vi "SendHRS.vi"(8 "error in (no error)":errorcluster, 10 "HRS data":u32[](array[numeric]), 11 "Database ref":refnum<k24>) -> (0 "error out":errorcluster)   [LabVIEW 2015]
uses:
  C:/Users/Bartek/Desktop/NORDIC Labview GUI/DLLs/NordicDatabaseDLL.dll
  DLLs/NordicDatabaseDLL.dll
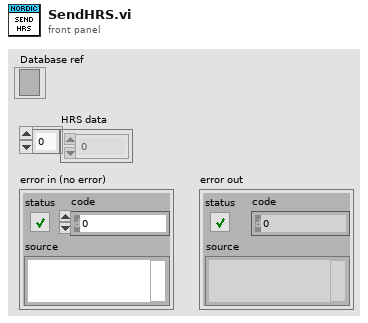
[diagram p1: front panel]
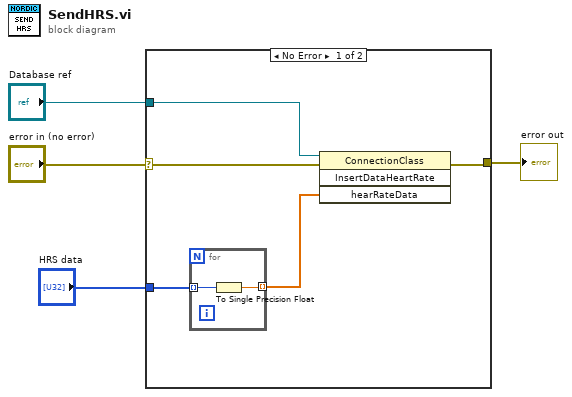
[diagram p0: block diagram]
diagram:
  n1 = case shown="No Error" "error in (no error)" {
    selector: "error in (no error)" -> [w8 w12]
    tunnel: [w5 w12] -> w3
    tunnel: "Database ref" -> [w9 _]
    tunnel: "HRS data" -> [w6 _]
    frame No Error {
      n2 = for {
        tunnel: [w11] -> w7 mode=indexing
        tunnel: w6 -> [w10] mode=indexing
        n3 = To Single Precision Float(number=w10) -> (single precision float=w11:sgl)
      }
      n4 = invoke class="ConnectionClass" method="InsertDataHeartRate"(reference=w9, error in=w8, "hearRateData"=w7) -> (error out=w5:errorcluster)  [unwired: 1 in, 3 out]
    }
    frame Error {
    }
  }
  "error out" <- w3
